vi "VeristandStop.vi"(8 "error in (no error)":errorcluster, 10 "CloseApp?":bool, 11 "CloseUIManager?":bool) -> (0 "error out":errorcluster)   [LabVIEW 2020, in "ni-veristand-steps-runtime-lib.lvlib"]
uses:
  ni-veristand-steps-runtime-lib.lvlib
  <vilib>/NI VeriStand/Execution/Project/NI_VS Project ExecutionAPI.lvlib
  <vilib>/NI VeriStand/Execution/Workspace/NI_VS Workspace ExecutionAPI.lvlib
panel:
  in  "stop":bool
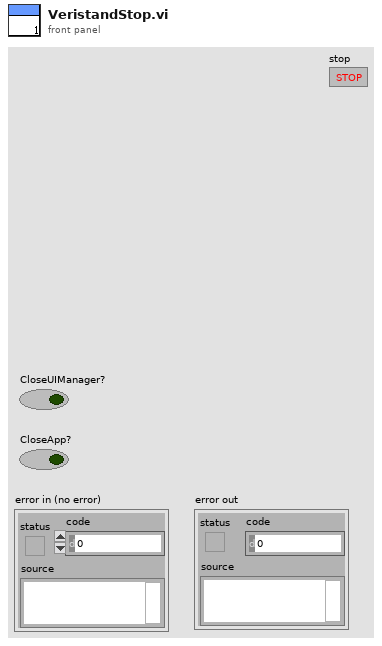
[diagram p1: front panel]
types:
  T1 = typedef "ni-veristand-steps-runtime-lib.lvlib/VeriStand dotNet References.ctl" = cluster{"ModelManager":T2, "AlarmManager":T3, "ChannelFault":T4, "WorkspaceManager":T5, "Project Ref":T6}
  T2 = typedef "NI_VS ModelManager ExecutionAPI.lvlib/ModelManagerAPI.ctl" = refnum<k24>
  T3 = typedef "NI_VS AlarmManager ExecutionAPI.lvlib/AlarmManagerAPI.ctl" = refnum<k24>
  T4 = typedef "NI_VS ChannelFault ExecutionAPI.lvlib/ChannelFaultAPI.ctl" = refnum<k24>
  T5 = typedef "NI_VS Workspace ExecutionAPI.lvlib/WorkspaceAPI.ctl" = refnum<k24>
  T6 = typedef "NI_VS Project ExecutionAPI.lvlib/Project Ref.ctl" = refnum<k24>
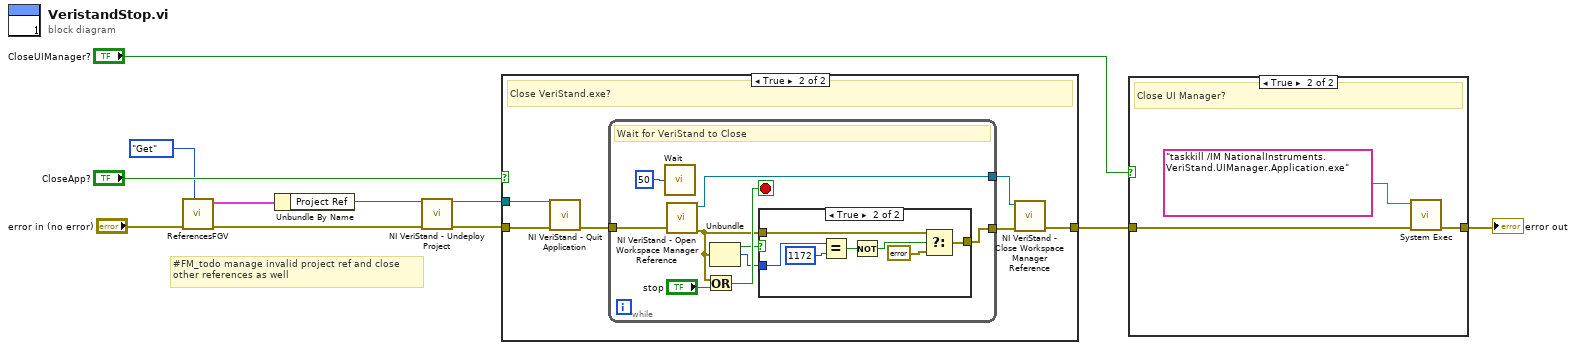
[diagram p0: block diagram]
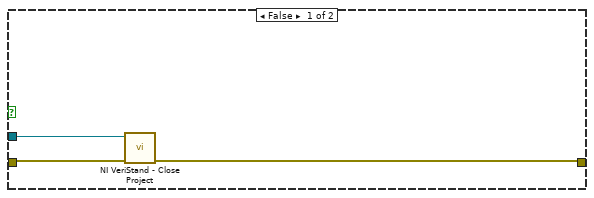
[diagram p3: hidden frame]
diagram:
  # "#FM_todo manage invalid project ref and close\nother references as well"
  n1 = call "ReferencesFGV.vi"("Get/Set"=enum16{"Get", "Set"}."Get", "error in (no error)"="error in (no error)") -> ("error out"=w8:errorcluster, "VeriStand dotNET Refs out"=w5:T1)  [unwired: 8 in]
  n2 = Unbundle By Name(w5) -> ("Project Ref"=w4:T6)
  n3 = call <vilib>:"NI VeriStand - Undeploy Project.vi"("error in (no error)"=w8, "Project Ref in"=w4) -> ("error out"=w10:errorcluster, "Project Ref out"=w9:T6)  [unwired: 8 in]
  n4 = case shown="True" "CloseApp?" {
    tunnel: w9 -> [w14 w20]
    tunnel: w10 -> [w13 w19]
    tunnel: [w12 w15] -> w2
    frame False {
      n5 = call <vilib>:"NI VeriStand - Close Project.vi"("error in (no error)"=w13, "Project Ref in"=w14) -> ("error out"=w12:errorcluster)  [unwired: 8 in, 1 out]
    }
    frame True {
      # "Close VeriStand.exe?"
      n6 = call <vilib>:"NI VeriStand - Quit Application.vi"("error in (no error)"=w19, "Project Ref in"=w20) -> ("error out"=w16:errorcluster)  [unwired: 8 in, 1 out]
      n7 = while {
        tunnel: [w29] -> w17
        tunnel: [w21] -> w18
        tunnel: w16 -> [w22]
        stop <- w27 stop-if-true
        # "Wait for VeriStand to Close"
        n8 = call "Wait"("Count(mSec)"=u32 50) -> ()  [unwired: 1 out]
        n9 = call <vilib>:"NI VeriStand - Open Workspace Manager Reference.vi"("error in (no error)"=w22) -> ("error out"=w23:errorcluster, "WorkspaceManager"=w29:T5)  [unwired: 9 in]
        n10 = Or(x=w23, y="stop") -> (x .or. y?=w27:bool)
        n11 = Unbundle(w23) -> ("status"=w25:bool, "code"=w24:i32)  [unwired: 1 out]
        n12 = case shown="True" w25 {
          tunnel: w24 -> [_ w37]
          tunnel: w23 -> [w30 w32]
          tunnel: [w30 w31] -> w21
          frame False {
          }
          frame True {
            n13 = Equal?(x=w37, y=1172) -> (x = y?=w35:bool)
            n14 = Not(x=w35) -> (.not. x?=w34:bool)
            n15 = Select(t=w32, s=w34, f=errorcluster {"status"=FALSE, "code"=0, "source"=""} ("error in (no error)")) -> (s? t:f=w31:errorcluster)
          }
        }
      }
      n16 = call <vilib>:"NI VeriStand - Close Workspace Manager Reference.vi"("error in (no error)"=w18, "WorkspaceManager"=w17) -> ("error out"=w15:errorcluster)  [unwired: 9 in]
    }
  }
  n17 = case shown="True" "CloseUIManager?" {
    tunnel: w2 -> [w38 w41]
    tunnel: [w38 w40] -> w1
    frame False {
    }
    frame True {
      # "Close UI Manager?"
      n18 = call <vilib>:"System Exec.vi"("error in (no error)"=w41, "command line"="taskkill /IM NationalInstruments.VeriStand.UIManager.Application.exe" ("standard input")) -> ("error out"=w40:errorcluster)  [unwired: 6 in, 3 out]
    }
  }
  "error out" <- w1
